vi "CH_LM Config Statistics Restart Mode.vi"(0 "Meter Index":i32, 2 "Restart Mode (f:manual)":bool, 5 "error in (no error)":errorcluster, 7 "Timeout / ms (3000)":i32=3000, 8 "Action (query)":bool, 9 "Lock Timeout / ms (1000)":i32=1000) -> (11 "Lock timed out":bool, 14 "Meter Index":i32, 16 "Restart Mode":bool, 19 "error out":errorcluster)   [LabVIEW 2012, in "CH_LM.lvlib"]
doc: "This command will select the action to be taken at the end of a statistical batch. Automatic will begin a new batch immediately upon logging the data from the previous batch.\n\n<B>Hint:</B> Manual will require the start signal (see CH_LM Config Statistics StartStop.vi)"
uses:
  CH_LM.lvlib
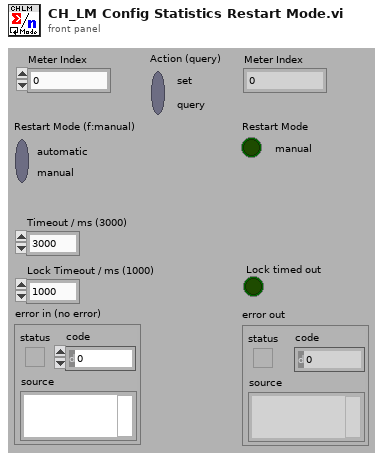
[diagram p1: front panel]
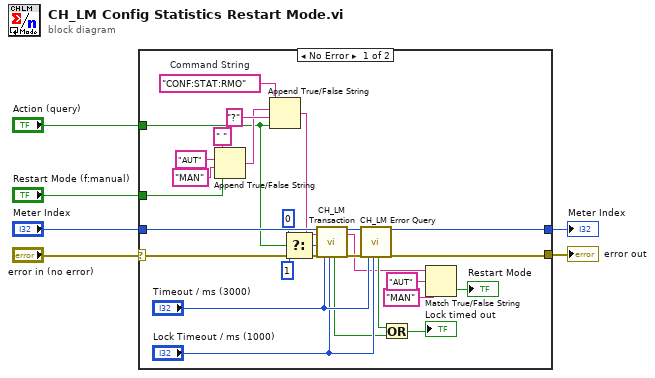
[diagram p0: block diagram]
diagram:
  n1 = case shown="No Error" "error in (no error)" {
    selector: "error in (no error)" -> [w33 w35]
    tunnel: [w31 w35] -> w6
    tunnel: "Meter Index" -> [w32 w34]
    tunnel: [w30 w34] -> w3
    tunnel: "Restart Mode (f:manual)" -> [w18 _]
    tunnel: "Action (query)" -> [w7 _]
    frame No Error {
      w11 = "CONF:STAT:RMO"  # Command String
      n2 = Append True/False String(1:w18, 2:"MAN" ("false string"), 3:"AUT" ("true string"), 4:" " ("string (\"\")")) -> (0:w9:string)
      n3 = Append True/False String(1:w7, 2:"?" ("false string"), 3:w9, 4:w11) -> (0:w8:string)
      n4 = Select(t=0, s=w7, f=1) -> (s? t:f=w20:i32)
      n5 = call "CH_LM Transaction.vi"("Meter Index"=w32, "Command String"=w8, "NofStrings (-1:all)"=w20, "error in (no error)"=w33, "Timeout / ms (3000)"="Timeout / ms (3000)", "Lock Timeout / ms (1000)"="Lock Timeout / ms (1000)") -> ("Lock timed out"=w24:bool, "Meter Index"=w27:i32, "Response"=w16:string, "error out"=w26:errorcluster)  [unwired: 10 out]
      n6 = call "CH_LM Error Query.vi"("Meter Index"=w27, "error in (no error)"=w26, "Timeout / ms (3000)"="Timeout / ms (3000)", "Lock Timeout / ms (1000)"="Lock Timeout / ms (1000)") -> ("Lock timed out"=w25:bool, "Meter Index"=w30:i32, "error out"=w31:errorcluster)  [unwired: 13 out]
      n7 = Or(x=w25, y=w24) -> (x .or. y?=→"Lock timed out":bool)
      n8 = Match True/False String(2:"MAN" ("false string"), 3:"AUT" ("true string"), 4:w16) -> (0:→"Restart Mode":bool)  [unwired: 1 out]
    }
    frame Error {
    }
  }
  "error out" <- w6
  "Meter Index" <- w3
